vi "Read-Write Measurement Settings File.vi"(0 "configuration file path":path=path "C:/ProgramData/PVI Systems/Staple Inspection System/Measurement Settings.xml", 1 "Measurement Settings":T2={"Image path"=path "J:/Staple Images/Reference Staples 2014-09-29/Under/1 staple 2014-09-26T17.36.27 Composite Focus.tif", "Image Paths"=[], "Index"=0, "AutoContinue"=FALSE, "Image Type"=0, "Image In"=refnum, "Image Dst"=refnum, "Pre-Rotate"=0.0, "Angle, OverCrimp"=[], "Inspect Backplane"=TRUE, "Inspect OverCrimp"=TRUE, "Inspect UnderCrimp"=TRUE, "Upsample to"=0.0, "All Dir"=path "", "Folders"=[], "Folder Index"=0, "Angle, OuterLine"=[], "Angle, InnerLine"=[], "Angle, UnderCrimp"=[], "Cal Img Path"=path "C:/Projects/codedepot/Covidien/2014-1011 Covidien Automated Staple Measurement/Images/calibration/Calibration 2014-08-22T12.12.45/Calibration Template.png", "Show Result Overall"=FALSE} {"Upsample to" min=0.0 max=4000.0 step=1.0; "Pre-Rotate" min=0.0 max=360.0 step=1.0; "Image Type" items=["Grayscale (U8)", "Grayscale (I16)", "Grayscale (SGL)", "Complex (CSG)", "RGB (U32)", "HSL (U32)", "RGB (U64)", "Grayscale (U16)"]}, 2 "Mode":T1=enum."Write", 3 "error in":errorcluster) -> (7 "Config File Path":path=path "C:/ProgramData/PVI Systems/Staple Inspection System/Config.ini", 8 "Measurement Settings":T2={"Image path"=path "J:/Staple Images/Reference Staples 2014-09-29/Under/1 staple 2014-09-26T17.36.27 Composite Focus.tif", "Image Paths"=[], "Index"=0, "AutoContinue"=FALSE, "Image Type"=0, "Image In"=refnum, "Image Dst"=refnum, "Pre-Rotate"=0.0, "Angle, OverCrimp"=[], "Inspect Backplane"=TRUE, "Inspect OverCrimp"=TRUE, "Inspect UnderCrimp"=TRUE, "Upsample to"=0.0, "All Dir"=path "", "Folders"=[], "Folder Index"=0, "Angle, OuterLine"=[], "Angle, InnerLine"=[], "Angle, UnderCrimp"=[], "Cal Img Path"=path "C:/Projects/codedepot/Covidien/2014-1011 Covidien Automated Staple Measurement/Images/calibration/Calibration 2014-08-22T12.12.45/Calibration Template.png", "Show Result Overall"=FALSE} {"Upsample to" min=0.0 max=4000.0 step=1.0; "Pre-Rotate" min=0.0 max=360.0 step=1.0; "Image Type" items=["Grayscale (U8)", "Grayscale (I16)", "Grayscale (SGL)", "Complex (CSG)", "RGB (U32)", "HSL (U32)", "RGB (U64)", "Grayscale (U16)"]}, 10 "error out":errorcluster)   [LabVIEW 2013, in "Config Module.lvlib"]
uses:
  Config Module.lvlib
  Measurement Library/Controls/ASMS-Settings Cluster.ctl
  <vilib>/vision/Image Controls.llb/IMAQ Image.ctl
  Controls/Config File Operation Enum.ctl
  XML Config/XML Config.lvlib
  Measurement Library/Measurement Library.lvlib
panel:
  out "XML":string
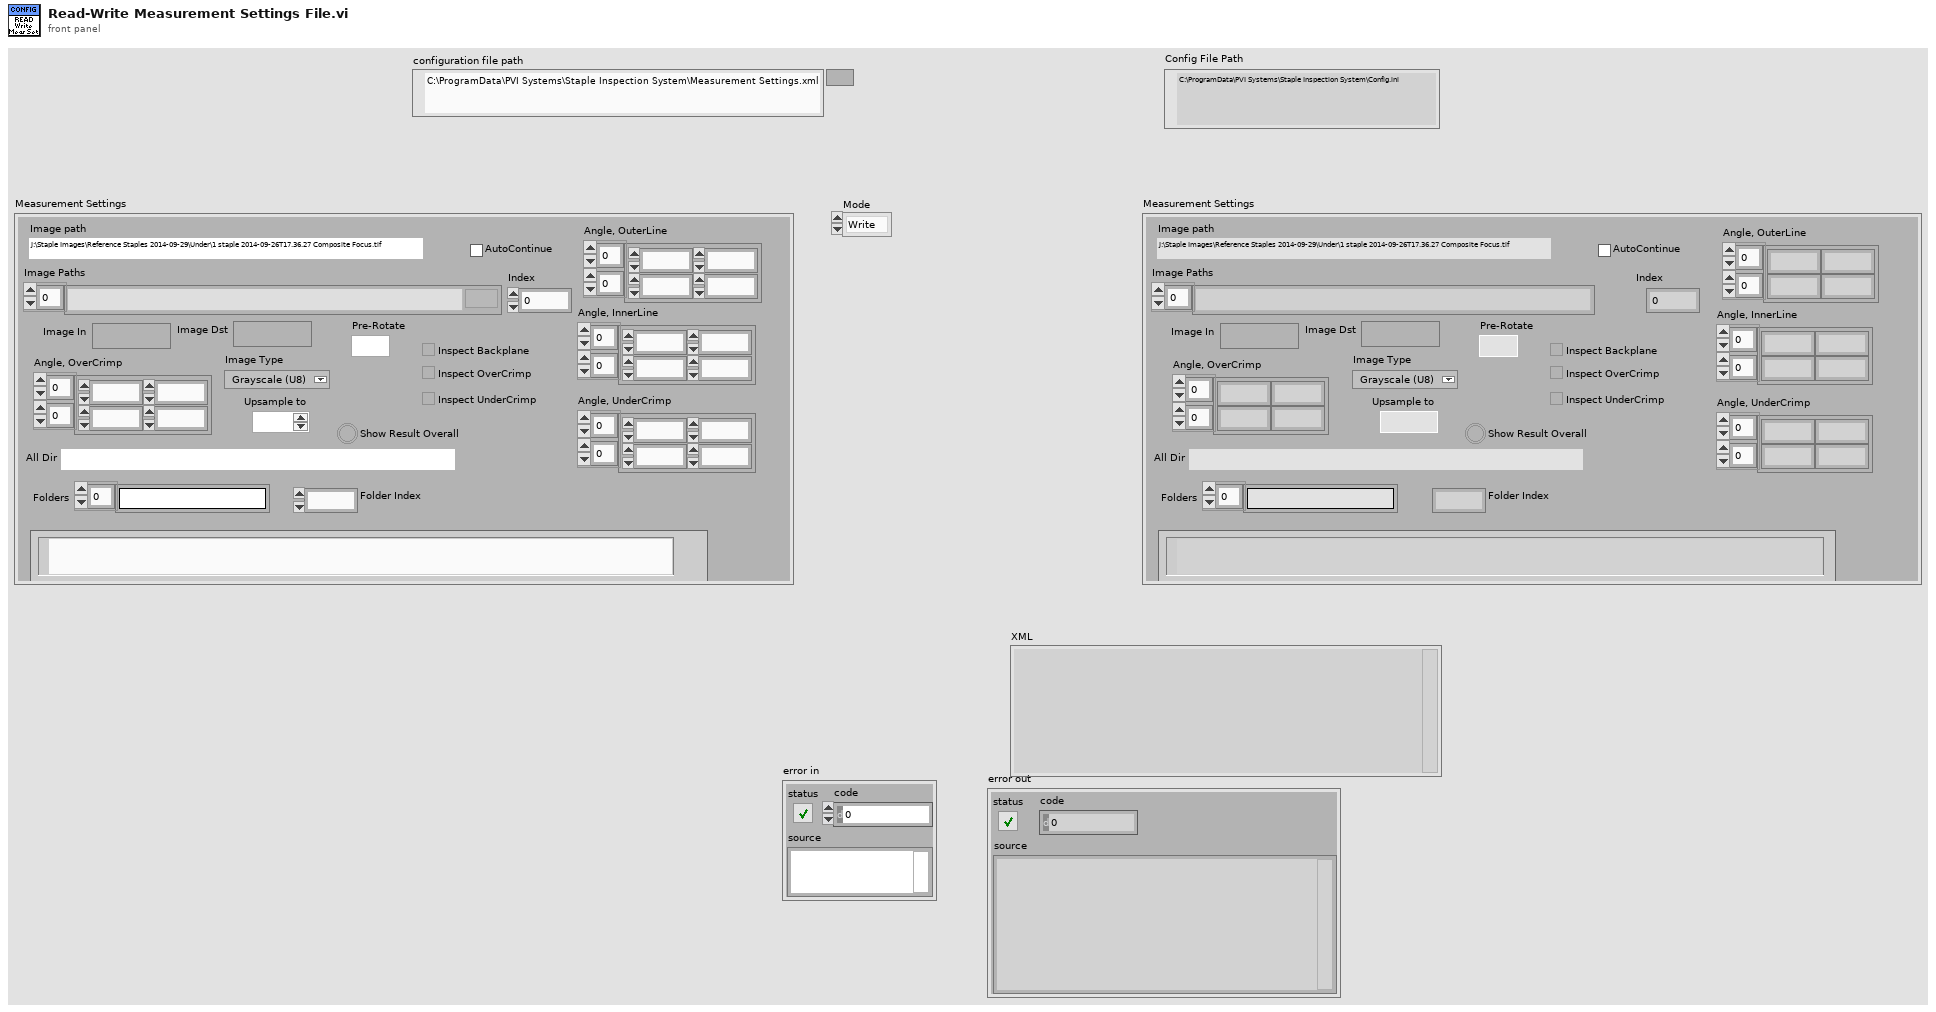
[diagram p1: front panel]
types:
  T1 = typedef "Config Module.lvlib/Config File Operation Enum.ctl" = enum16{"Read", "Write"}
  T2 = typedef "Measurement Library.lvlib/ASMS-Settings Cluster.ctl" = cluster{"Image path":path, "Image Paths":path[], "Index":u32, "AutoContinue":bool, "Image Type":T3, "Image In":T4, "Image Dst":T4, "Pre-Rotate":dbl, "Angle, OverCrimp":dbl[][], "Inspect Backplane":bool, "Inspect OverCrimp":bool, "Inspect UnderCrimp":bool, "Upsample to":dbl, "All Dir":path, "Folders":string[], "Folder Index":u32, "Angle, OuterLine":dbl[][], "Angle, InnerLine":dbl[][], "Angle, UnderCrimp":dbl[][], "Cal Img Path":path, "Show Result Overall":bool}
  T3 = typedef "Image Type" = u32
  T4 = typedef "IMAQ Image.ctl" = refnum<image>
  T5 = enum16{"open", "replace", "create", "open or create", "replace or create", "replace or create with confirmation"}
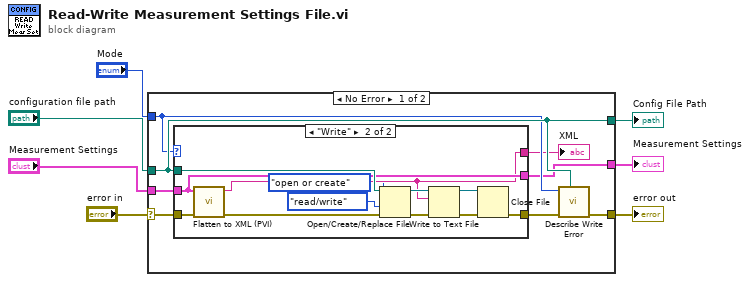
[diagram p0: block diagram]
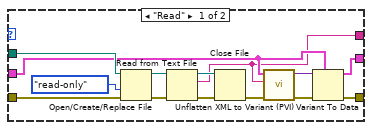
[diagram p2: hidden frame]
diagram:
  n1 = case shown="No Error" "error in" {
    selector: "error in" -> [w14 w43]
    tunnel: [w15 w43] -> w7
    tunnel: "configuration file path" -> [w13 w44]
    tunnel: "Measurement Settings" -> [w11 w42]
    tunnel: [w13 w44] -> w6
    tunnel: "Mode" -> [w12 _]
    tunnel: [w8 w42] -> w3
    frame No Error {
      n2 = case shown="\"Write\"" w12 {
        tunnel: w14 -> [w29 w36]
        tunnel: w13 -> [w24 w41]
        tunnel: w11 -> [w20 w37]
        tunnel: [w18 w34] -> w10
        tunnel: [w17 w31] -> w9
        tunnel: [w16 w37] -> w8
        frame "Read" {
          n3 = Open/Create/Replace File(file path (use dialog)=w24, error in=w29, access (0:read/write)=enum16{"read/write", "read-only", "write-only"}."read-only") -> (refnum out=w26:refnum<file>, error out=w28:errorcluster)  [unwired: 3 in, 1 out]
          n4 = Read from Text File(file (use dialog)=w26, error in=w28) -> (refnum out=w25:refnum<file>, text=w18:string, error out=w27:errorcluster)  [unwired: 2 in, 1 out]
          n5 = Close File(refnum=w25, error in=w27) -> (error out=w22:errorcluster)  [unwired: 1 out]
          n6 = call "Unflatten XML to Variant (PVI).vi"("error in (no error)"=w22, "XML"=w18, "Variant in (for type and default data)"=w20) -> ("error out"=w19:errorcluster, "Variant out"=w21:variant)  [unwired: 7 in]
          n7 = Variant To Data(error in=w19, type=w20, Variant=w21) -> (data=w16:T2, error out=w17:errorcluster)
        }
        frame "Write" {
          n8 = call "Flatten to XML (PVI).vi"("error in (no error)"=w36, "Variant"=w37) -> ("error out"=w35:errorcluster, "XML"=w34:string)  [unwired: 8 in]
          n9 = Open/Create/Replace File(file path (use dialog)=w41, error in=w35, operation (0:open)=T5."open or create", access (0:read/write)=enum16{"read/write", "read-only", "write-only"}."read/write") -> (refnum out=w39:refnum<file>, error out=w38:errorcluster)  [unwired: 2 in, 1 out]
          n10 = Write to Text File(file (use dialog)=w39, text=w34, error in=w38) -> (refnum out=w33:refnum<file>, error out=w32:errorcluster)  [unwired: 1 in, 1 out]
          n11 = Close File(refnum=w33, error in=w32) -> (error out=w31:errorcluster)  [unwired: 1 out]
        }
      }
      "XML" <- w10
      n12 = call "Describe Write Error.vi"("Config File Path"=w13, "error in (no error)"=w9, "Mode"=w12) -> ("error out"=w15:errorcluster)  [unwired: 8 in]
    }
    frame Error {
    }
  }
  "error out" <- w7
  "Config File Path" <- w6
  "Measurement Settings" <- w3
